vi "Concatenate.vi"() -> ()   [LabVIEW 2024]
panel:
  out "length 2":i32
  out "length":i32
  out "concatenated string":string
  in  "String 2":string
  in  "String 1":string
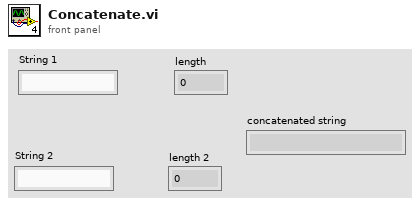
[diagram p1: front panel]
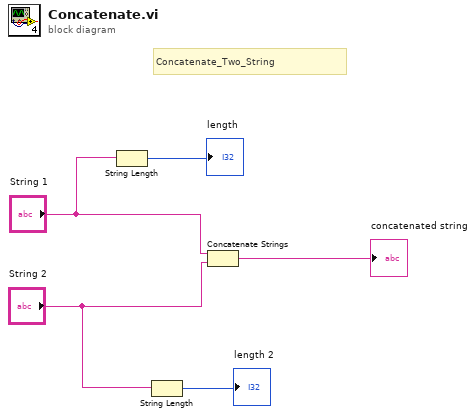
[diagram p0: block diagram]
diagram:
  # "Concatenate_Two_String"
  n1 = String Length(string="String 1") -> (length=→"length":i32)
  n2 = String Length(string="String 2") -> (length=→"length 2":i32)
  n3 = Concatenate Strings("String 1", "String 2") -> (→"concatenated string":string)
